vi "Set Channel Value.vi"(8 "error in":errorcluster, 9 "Value":dbl format="%#_13g", 10 "Data Reference in":T1 format="%.0x", 11 "VS Engine Interface in":refnum<class "VS Engine Interface.lvclass">) -> (0 "error out":errorcluster, 3 "VS Engine Interface out":refnum<class "VS Engine Interface.lvclass">)   [LabVIEW 2024, in "VS Engine Abstraction.lvlib" / "VS Engine Interface.lvclass"]
uses:
  VS Engine Interface.lvclass
  <vilib>/NI VeriStand/Custom Device API/Data Reference.ctl
  <vilib>/NI VeriStand/Custom Device API/Custom Device API.lvlib
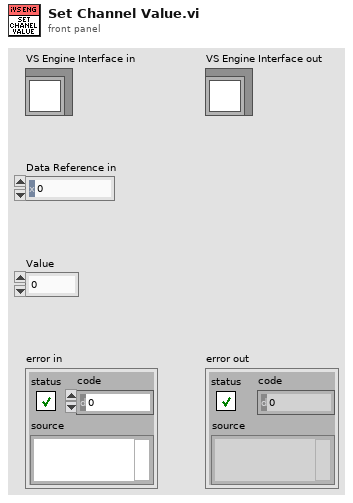
[diagram p1: front panel]
types:
  T1 = typedef "Custom Device API.lvlib/Data Reference.ctl" = i32
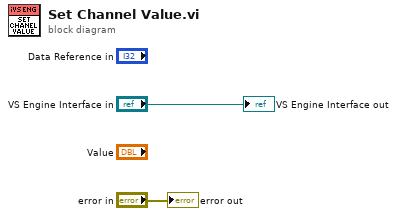
[diagram p0: block diagram]
diagram:
  "error out" <- "error in"
  "VS Engine Interface out" <- "VS Engine Interface in"
